vi "SLSC Get IP Address from Chassis.vi"(8 "error in (no error)":errorcluster, 10 "IP Address Global Name":string, 11 "Node Ptr":T1 format="%.0x") -> (0 "error out":errorcluster, 1 "Chassis ID Type":i32(ring) items=["ChassisName", "HostnameIPAddress"], 2 "Name or IP Address":string, 3 "Node Ptr":T1 format="%.0x", 4 "Password":string, 5 "Username":string)   [LabVIEW 2017, in "SLSC CD System Explorer.lvlib"]
uses:
  SLSC CD System Explorer.lvlib
  <vilib>/NI Veristand/Custom Device API/Custom Device Item Ref.ctl
  NationalInstruments.VeriStand.SystemDefinitionAPI
  <vilib>/NI Veristand/Custom Device API/Custom Device API.lvlib
  <vilib>/NI Veristand/Custom Device API/Get Item Property (String).vi
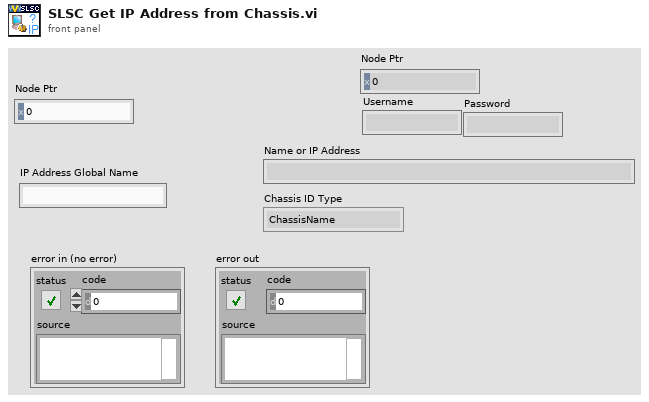
[diagram p1: front panel]
types:
  T1 = typedef "Custom Device API.lvlib/Custom Device Item Ref.ctl" = u64
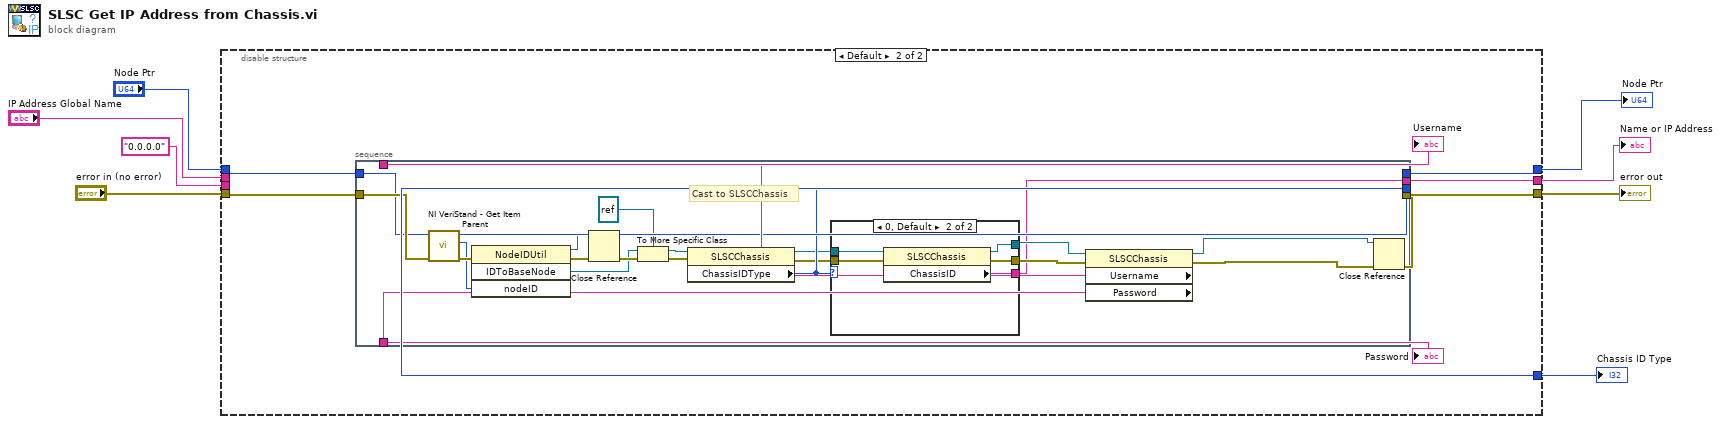
[diagram p0: block diagram]
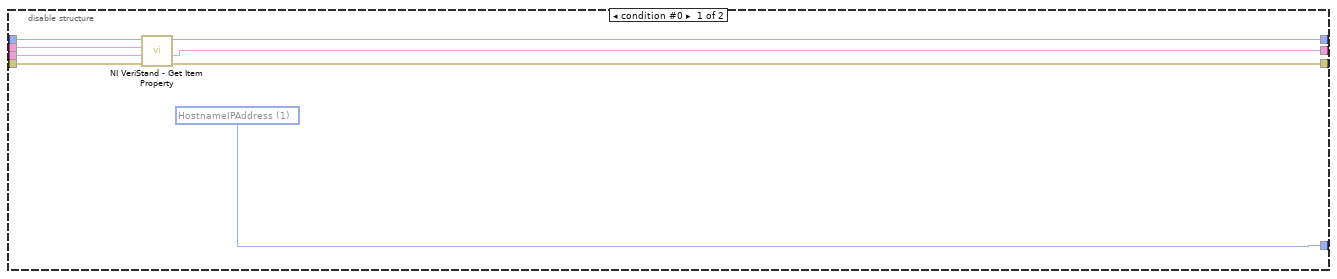
[diagram p2: hidden frame]
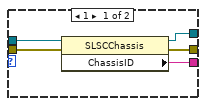
[diagram p3: hidden frame]
diagram:
  n1 = disable-structure shown="Default" {
    disable-tunnel: [w16 w21] -> w8
    disable-tunnel: [w15 w20] -> w7
    disable-tunnel: "0.0.0.0" ("Default Value") -> [w14 _]
    disable-tunnel: "Node Ptr" -> [w13 w24]
    disable-tunnel: "error in (no error)" -> [w12 w23]
    disable-tunnel: [w11 w22] -> w3
    disable-tunnel: "IP Address Global Name" -> [w10 _]
    disable-tunnel: [w9 w19] -> w1
    frame condition #0 {
      w9 = 1 items=["ChassisName", "HostnameIPAddress"] ("ChassisIDType")
      n2 = call-poly <vilib>:"NI VeriStand - Get Item Property.vi"("error in (no error)"=w12, "Default Value"=w14, "Property Name"=w10, "Item Ref in"=w13) -> ("error out"=w15:errorcluster, "Value"=w16:string, "Item Ref out"=w11:T1)  [unwired: 4 in, 1 out]
    }
    frame condition #1 (active) {
      n3 = stacked-sequence {
        tunnel: [w34] -> w20
        tunnel: [w40] -> w19
        tunnel: [w28] -> w21
        tunnel: [w41] -> w22
        tunnel: [w47] -> w17
        tunnel: [w46] -> w18
        tunnel: w23 -> [w35]
        tunnel: w24 -> [w26]
        frame #0 {
          # "Cast to SLSCChassis"
          n4 = call <vilib>:"NI VeriStand - Get Item Parent.vi"("error in (no error)"=w35, "Item Ref in"=w26) -> ("error out"=w27:errorcluster, "Parent Ref"=w25:T1, "Item Ref out"=w41:T1)  [unwired: 6 in, 1 out]
          n5 = invoke class="NodeIDUtil" method="IDToBaseNode"(error in=w27, "nodeID"=w25) -> (reference out=w33:refnum<k24>, error out=w32:errorcluster, "IDToBaseNode"=w30:refnum<k24>)  [unwired: 2 in, 1 out]
          n6 = Close Reference(reference=w33, error in (no error)=w32) -> (error out=w31:errorcluster)
          n7 = To More Specific Class(target class=refnum<k24> refnum, reference=w30, error in=w31) -> (specific class reference=w36:refnum<k24>, error out=w37:errorcluster)
          n8 = property class="SLSCChassis"(reference=w36, error in=w37) -> (reference out=w38:refnum<k24>, error out=w39:errorcluster, "ChassisIDType"=w40:i32)
          n9 = case shown="0, Default" w40 {
            tunnel: [w52 w57] -> w28
            tunnel: w38 -> [w51 w56]
            tunnel: w39 -> [w50 w55]
            tunnel: [w49 w54] -> w42
            tunnel: [w48 w53] -> w43
            frame 1 {
              n10 = property class="SLSCChassis"(reference=w51, error in=w50) -> (reference out=w49:refnum<k24>, error out=w48:errorcluster, "ChassisID"=w52:string)
            }
            frame 0, Default {
              n11 = property class="SLSCChassis"(reference=w56, error in=w55) -> (reference out=w54:refnum<k24>, error out=w53:errorcluster, "ChassisID"=w57:string)
            }
          }
          n12 = property class="SLSCChassis"(reference=w42, error in=w43) -> (reference out=w44:refnum<k24>, error out=w45:errorcluster, "Username"=w46:string, "Password"=w47:string)
          n13 = Close Reference(reference=w44, error in (no error)=w45) -> (error out=w34:errorcluster)
        }
      }
      "Username" <- w18
      "Password" <- w17
    }
  }
  "Name or IP Address" <- w8
  "error out" <- w7
  "Node Ptr" <- w3
  "Chassis ID Type" <- w1
